vi "Write.vi"(7 "error in (no error)":errorcluster, 9 "Values":dbl[](array[numeric]), 10 "AO Ref In":T1) -> (0 "error out":errorcluster, 3 "AO Ref Out":T1)   [LabVIEW 2021, in "AO.lvlib"]
doc: "Writes values to one or more analog output channels."
uses:
  <vilib>/myRIO/Instrument Drivers/Onboard IO/AO/AO.lvlib
  <vilib>/myRIO/Instrument Drivers/Onboard IO/AO/typedefs/AO Reference.ctl
  <vilib>/myRIO/Common/Instrument Driver Framework/Utilities/typedefs/myRIO Generic Hardware Reference.ctl
  <vilib>/myRIO/Common/Instrument Driver Framework/Utilities/typedefs/Hardware Version Enum.ctl
  <vilib>/myRIO/Common/Instrument Driver Framework/Utilities/typedefs/myRIO v1.0 Reference.ctl
  <vilib>/myRIO/Common/Instrument Driver Framework/Utilities/typedefs/Generic FPGA Reference.ctl
  <vilib>/myRIO/Common/Instrument Driver Framework/myRIO v1.0/AO/typedefs/AO Channels List.ctl
  <vilib>/myRIO/Common/Instrument Driver Framework/myRIO v1.0/AO/typedefs/AO Channels Enum.ctl
  <vilib>/myRIO/Common/Instrument Driver Framework/Utilities/typedefs/Analog Scaling Constants List.ctl
  <vilib>/myRIO/Common/Instrument Driver Framework/Utilities/typedefs/Analog Scaling Constants.ctl
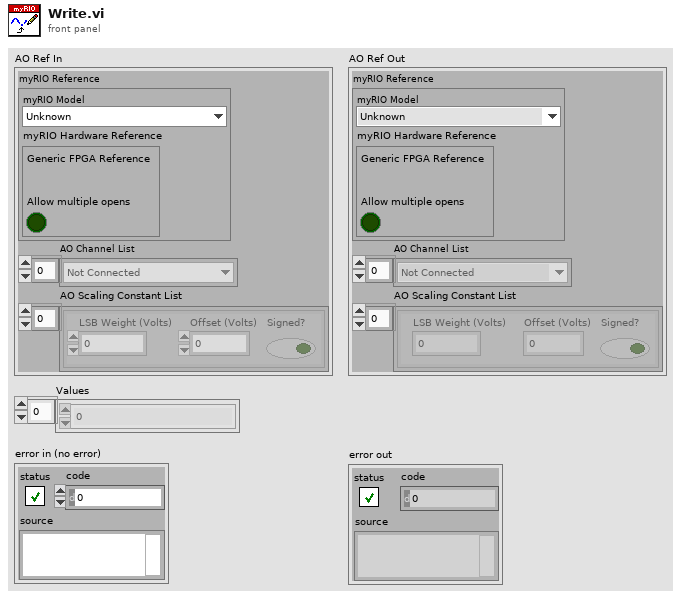
[diagram p1: front panel]
types:
  T1 = typedef "AO.lvlib/AO Reference.ctl" = cluster{"myRIO Reference":T2, "AO Channel List":T6, "AO Scaling Constant List":T8}
  T2 = typedef "myRIO Generic Hardware Reference.ctl" = cluster{"myRIO Model":T3, "myRIO Hardware Reference":T4}
  T3 = typedef "Hardware Version Enum.ctl" = enum16{"Unknown", "myRIO-1900", "myRIO-1950", "roboRIO", "NI ELVIS RIO CM", "ELVIS III"}
  T4 = typedef "myRIO v1.0 Reference.ctl" = cluster{"Generic FPGA Reference":T5, "Allow multiple opens":bool}
  T5 = typedef "Generic FPGA Reference.ctl" = refnum<k20>
  T6 = typedef "AO Channels List.ctl" = T7[]
  T7 = typedef "AO Channels Enum.ctl" = enum16{"Not Connected", "AudioOut/Left", "AudioOut/Right", "C/AO0", "C/AO1", "A/AO0", "A/AO1", "B/AO0", "B/AO1"}
  T8 = typedef "Analog Scaling Constants List.ctl" = T9[]
  T9 = typedef "Analog Scaling Constants.ctl" = cluster{"LSB Weight (Volts)":dbl, "Offset (Volts)":dbl, "Signed?":bool}
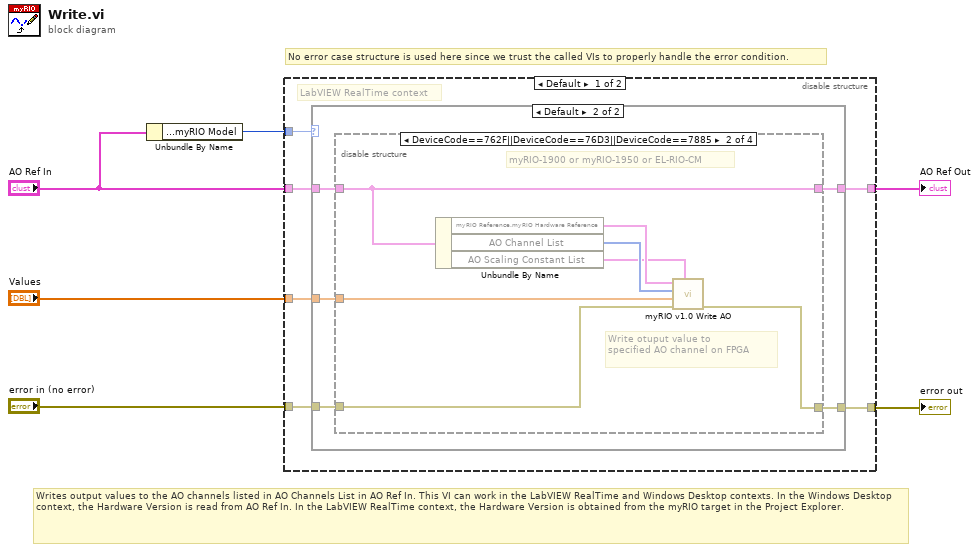
[diagram p0: block diagram]
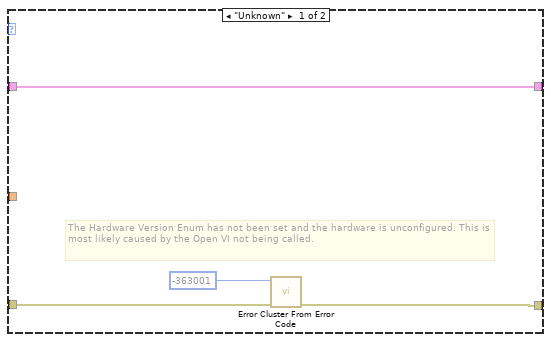
[diagram p2: hidden frame]
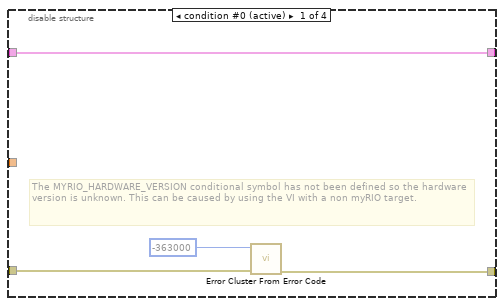
[diagram p3: hidden frame]
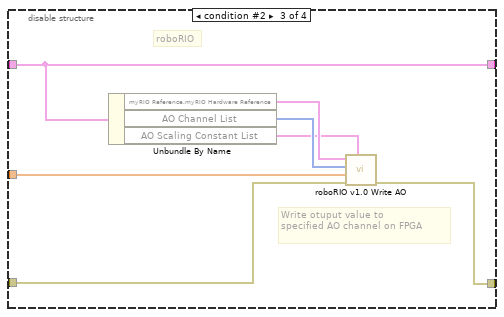
[diagram p4: hidden frame]
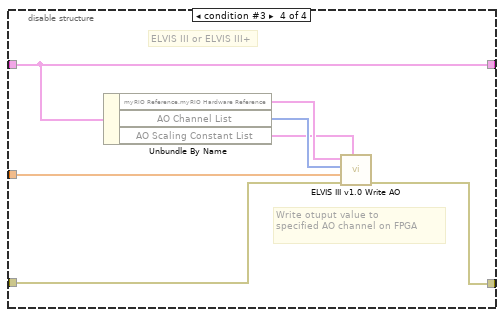
[diagram p5: hidden frame]
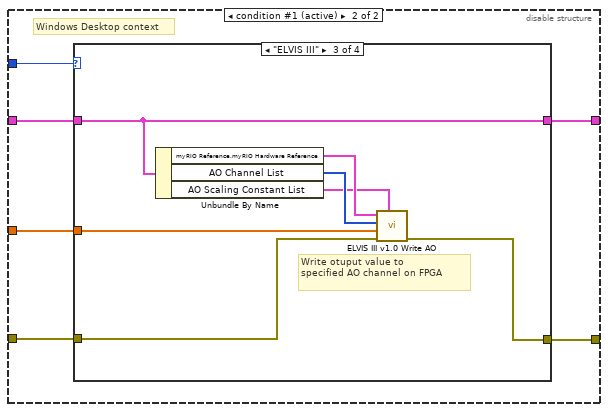
[diagram p6: hidden frame]
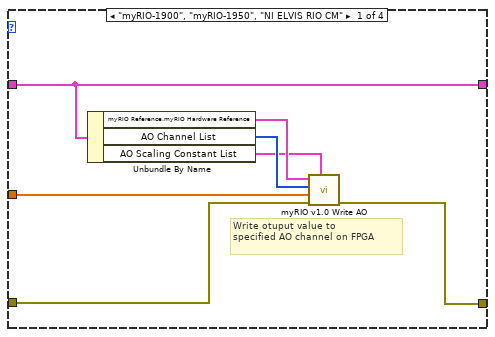
[diagram p7: hidden frame]
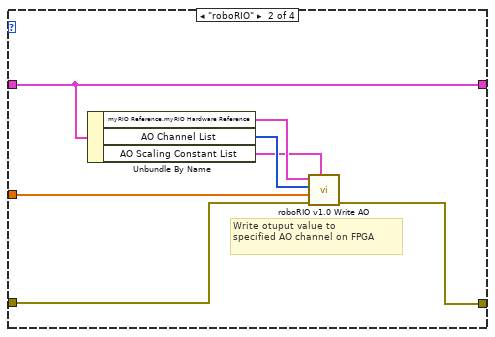
[diagram p8: hidden frame]
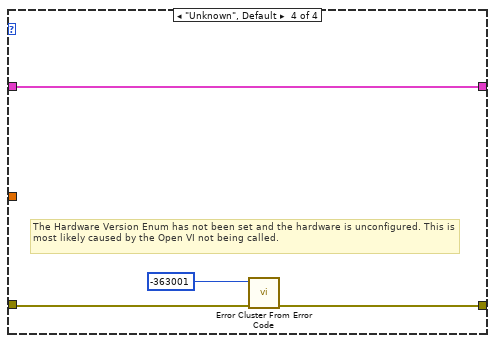
[diagram p9: hidden frame]
diagram:
  # "No error case structure is used here since we trust the called VIs to properly handle the error condition."
  # "Writes output values to the AO channels listed in AO Channels List in AO Ref In. This VI can work in the LabVIEW RealTime and Windows Desktop contexts. In the Windows Desktop context, the Hardware Version is read from AO Ref In. In the LabVIEW RealTime context, the Hardware Version is obtained from the myRIO target in the Project Explorer."
  n1 = Unbundle By Name("AO Ref In") -> ("myRIO Reference.myRIO Model"=w1:T3)
  n2 = disable-structure shown="Default" {
    disable-tunnel: [w12 w52] -> w3
    disable-tunnel: "AO Ref In" -> [w11 w49]
    disable-tunnel: "error in (no error)" -> [w10 w51]
    disable-tunnel: [w9 w50] -> w4
    disable-tunnel: "Values" -> [w8 w48]
    disable-tunnel: w1 -> [w7 w47]
    frame condition #0 {
      # "LabVIEW RealTime context"
      n3 = case shown="Default" w7 {
        tunnel: [w15 w21] -> w12
        tunnel: w11 -> [w13 w20]
        tunnel: w10 -> [w14 w19]
        tunnel: [w13 w18] -> w9
        tunnel: w8 -> [_ w17]
        frame "Unknown" {
          # "The Hardware Version Enum has not been set and the hardware is unconfigured. This is most likely caused by the Open VI not being called."
          n4 = call <vilib>:"Error Cluster From Error Code.vi"("error in (no error)"=w14, "error code (0)"=-363001) -> ("error out"=w15:errorcluster)  [unwired: 7 in]
        }
        frame Default {
          n5 = disable-structure shown="DeviceCode==762F||DeviceCode==76D3||DeviceCode==7885" {
            disable-tunnel: w20 -> [w22 w32 w39 w41]
            disable-tunnel: [w25 w29 w36 w40] -> w21
            disable-tunnel: w19 -> [w23 w31 w38 w42]
            disable-tunnel: [w22 w32 w39 w41] -> w18
            disable-tunnel: w17 -> [_ w28 w35 w43]
            frame condition #0 (active) {
              # "The MYRIO_HARDWARE_VERSION conditional symbol has not been defined so the hardware version is unknown. This can be caused by using the VI with a non myRIO target."
              n6 = call <vilib>:"Error Cluster From Error Code.vi"("error in (no error)"=w23, "error code (0)"=-363000) -> ("error out"=w25:errorcluster)  [unwired: 7 in]
            }
            frame condition #1 {
              # "myRIO-1900 or myRIO-1950 or EL-RIO-CM"
              # "Write otuput value to \nspecified AO channel on FPGA"
              n7 = Unbundle By Name(w32) -> ("myRIO Reference.myRIO Hardware Reference"=w27:T4, "AO Channel List"=w30:T6, "AO Scaling Constant List"=w26:T8)
              n8 = call <vilib>:"myRIO v1.0 Write AO.vi"("Scale Constants Array"=w26, "error in (no error)"=w31, "dbl Scaled Value List"=w28, "Channel List"=w30, "myRIO Ref In"=w27) -> ("error out"=w29:errorcluster)  [unwired: 5 in, 1 out]
            }
            frame condition #2 {
              # "roboRIO"
              # "Write otuput value to \nspecified AO channel on FPGA"
              n9 = Unbundle By Name(w39) -> ("myRIO Reference.myRIO Hardware Reference"=w34:T4, "AO Channel List"=w37:T6, "AO Scaling Constant List"=w33:T8)
              n10 = call <vilib>:"roboRIO v1.0 Write AO.vi"("Scale Constants Array"=w33, "error in (no error)"=w38, "dbl Scaled Value List"=w35, "Channel List"=w37, "myRIO Ref In"=w34) -> ("error out"=w36:errorcluster)  [unwired: 5 in, 1 out]
            }
            frame condition #3 {
              # "ELVIS III or ELVIS III+"
              # "Write otuput value to \nspecified AO channel on FPGA"
              n11 = Unbundle By Name(w41) -> ("myRIO Reference.myRIO Hardware Reference"=w45:T4, "AO Channel List"=w46:T6, "AO Scaling Constant List"=w44:T8)
              n12 = call <vilib>:"ELVIS III v1.0 Write AO.vi"("Scale Constants Array"=w44, "error in (no error)"=w42, "dbl Scaled Value List"=w43, "Channel List"=w46, "myRIO Ref In"=w45) -> ("error out"=w40:errorcluster)  [unwired: 5 in, 1 out]
            }
          }
        }
      }
    }
    frame condition #1 (active) {
      # "Windows Desktop context"
      n13 = case shown="\"ELVIS III\"" w47 {
        tunnel: [w56 w63 w68 w77] -> w52
        tunnel: w49 -> [w59 w66 w67 w74]
        tunnel: w51 -> [w57 w64 w69 w75]
        tunnel: [w59 w66 w67 w74] -> w50
        tunnel: w48 -> [w55 w62 w70 _]
        frame "myRIO-1900", "myRIO-1950", "NI ELVIS RIO CM" {
          # "Write otuput value to \nspecified AO channel on FPGA"
          n14 = Unbundle By Name(w59) -> ("myRIO Reference.myRIO Hardware Reference"=w54:T4, "AO Channel List"=w58:T6, "AO Scaling Constant List"=w53:T8)
          n15 = call <vilib>:"myRIO v1.0 Write AO.vi"("Scale Constants Array"=w53, "error in (no error)"=w57, "dbl Scaled Value List"=w55, "Channel List"=w58, "myRIO Ref In"=w54) -> ("error out"=w56:errorcluster)  [unwired: 5 in, 1 out]
        }
        frame "roboRIO" {
          # "Write otuput value to \nspecified AO channel on FPGA"
          n16 = Unbundle By Name(w66) -> ("myRIO Reference.myRIO Hardware Reference"=w61:T4, "AO Channel List"=w65:T6, "AO Scaling Constant List"=w60:T8)
          n17 = call <vilib>:"roboRIO v1.0 Write AO.vi"("Scale Constants Array"=w60, "error in (no error)"=w64, "dbl Scaled Value List"=w62, "Channel List"=w65, "myRIO Ref In"=w61) -> ("error out"=w63:errorcluster)  [unwired: 5 in, 1 out]
        }
        frame "ELVIS III" {
          # "Write otuput value to \nspecified AO channel on FPGA"
          n18 = Unbundle By Name(w67) -> ("myRIO Reference.myRIO Hardware Reference"=w72:T4, "AO Channel List"=w73:T6, "AO Scaling Constant List"=w71:T8)
          n19 = call <vilib>:"ELVIS III v1.0 Write AO.vi"("Scale Constants Array"=w71, "error in (no error)"=w69, "dbl Scaled Value List"=w70, "Channel List"=w73, "myRIO Ref In"=w72) -> ("error out"=w68:errorcluster)  [unwired: 5 in, 1 out]
        }
        frame "Unknown", Default {
          # "The Hardware Version Enum has not been set and the hardware is unconfigured. This is most likely caused by the Open VI not being called."
          n20 = call <vilib>:"Error Cluster From Error Code.vi"("error in (no error)"=w75, "error code (0)"=-363001) -> ("error out"=w77:errorcluster)  [unwired: 7 in]
        }
      }
    }
  }
  "AO Ref Out" <- w4
  "error out" <- w3
